vi "Write Data Type.vi"(8 "error in (no error)":errorcluster, 10 "Abs_String.lvclass":refnum<class "Abs_String.lvclass">, 11 "OnChange_Boolean in":refnum<class "OnChangeNotifier_String.lvclass">) -> (0 "error out":errorcluster, 3 "OnChange_Boolean out":refnum<class "OnChangeNotifier_String.lvclass">)   [LabVIEW 2021, in "OnChangeNotifier_String.lvclass"]
uses:
  OnChangeNotifier_String.lvclass
  <vilib>/TSA/Abstract Data Classes/Abs_Types/String/Abs_String.lvclass
  OnChangeNotifier_String.lvclass/OnChangeNotifier_String.ctl
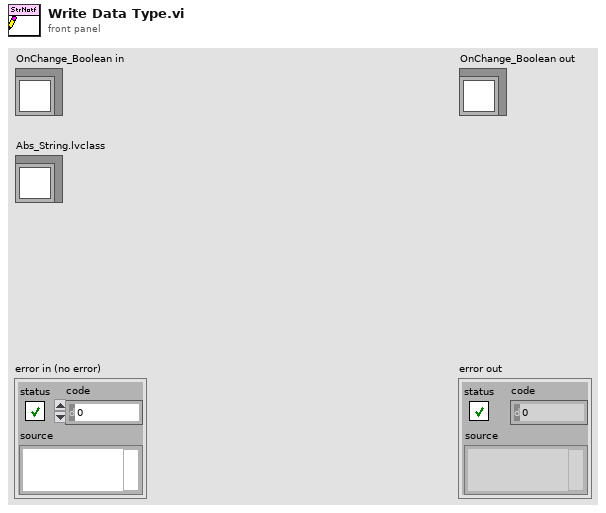
[diagram p1: front panel]
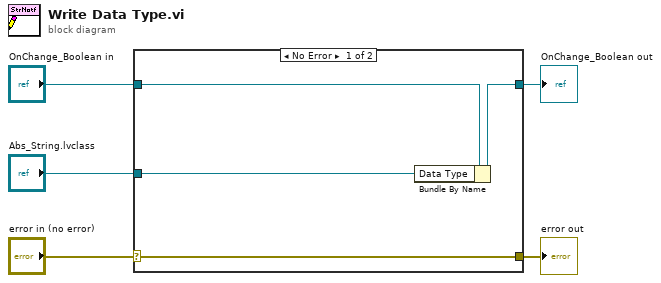
[diagram p0: block diagram]
diagram:
  n1 = case shown="No Error" "error in (no error)" {
    selector: "error in (no error)" -> [w9 w10]
    tunnel: [w9 w10] -> w4
    tunnel: [w7 w11] -> w2
    tunnel: "OnChange_Boolean in" -> [w8 w11]
    tunnel: "Abs_String.lvclass" -> [w6 _]
    frame No Error {
      n2 = Bundle By Name(cluster=w8, "Data Type"=w6) -> (w7:refnum<class "OnChangeNotifier_String.lvclass">)
    }
    frame Error {
    }
  }
  "error out" <- w4
  "OnChange_Boolean out" <- w2
